vi "find location.vi"(10 "Location Description":string, 11 "Defualt Device":T2 {"List of locations"."Position"."Position Y" format="%#.3f"; "List of locations"."Position"."Position X" format="%#.3f"}) -> (1 "Index of location":i32, 2 "Found?":bool, 3 "Location of input":T1 {"Position"."Position Y" format="%#.3f"; "Position"."Position X" format="%#.3f"})   [LabVIEW 2017]
uses:
  device.ctl
  location.ctl
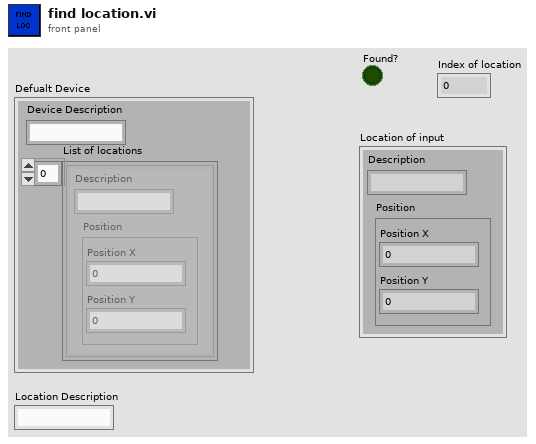
[diagram p1: front panel]
types:
  T1 = typedef "location.ctl" = cluster{"Description":string, "Position":cluster{"Position X":dbl, "Position Y":dbl}}
  T2 = typedef "device.ctl" = cluster{"List of locations":T1[], "Device Description":string}
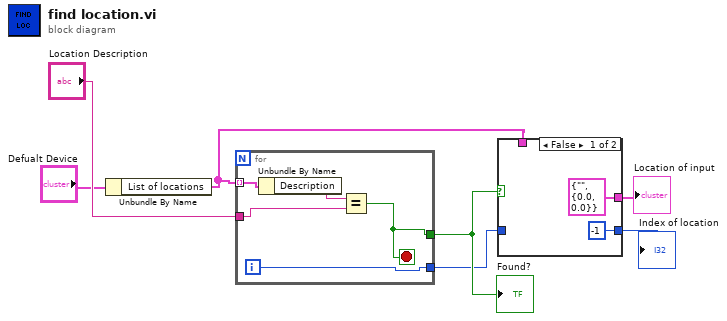
[diagram p0: block diagram]
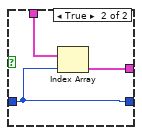
[diagram p2: hidden frame]
diagram:
  n1 = Unbundle By Name("Defualt Device") -> ("List of locations"=w4:T1[])
  n2 = for {
    tunnel: w4 -> [w9] mode=indexing
    tunnel: "Location Description" -> [w11]
    tunnel: [w10] -> w5
    tunnel: [w8] -> w3
    i -> [w8]
    stop <- w10 stop-if-true
    n3 = Unbundle By Name(w9) -> ("Description"=w12:string)
    n4 = Equal?(x=w12, y=w11) -> (x = y?=w10:bool)
  }
  "Found?" <- w5
  n5 = case shown="False" w5 {
    tunnel: w4 -> [_ w17]
    tunnel: w3 -> [_ w15]
    tunnel: [T1 {"Description"="", "Position"={"Position X"=0.0, "Position Y"=0.0}} ("Location of input") w16] -> w2
    tunnel: [-1 w15] -> w1
    frame False {
    }
    frame True {
      n6 = Index Array(array=w17, index=w15) -> (element=w16:T1)
    }
  }
  "Location of input" <- w2
  "Index of location" <- w1
